vi "GetConfigChain.vi"(8 "error in (no error)":errorcluster, 11 "reference in":refnum<class "Frequency_Counter_BK.lvclass">) -> (0 "error out":errorcluster, 2 "Config out":string[](array[string]), 3 "reference out":refnum<class "Frequency_Counter_BK.lvclass">)   [LabVIEW 2022 SP3, in "Frequency_Counter_BK.lvlib" / "Frequency_Counter_BK.lvclass"]
uses:
  Frequency_Counter_BK.lvclass
  Components/Frequency_Counter_Base.lvlibp/Frequency_Counter_Base.lvclass
  Components/ViPER.lvlibp/ViPER.lvclass
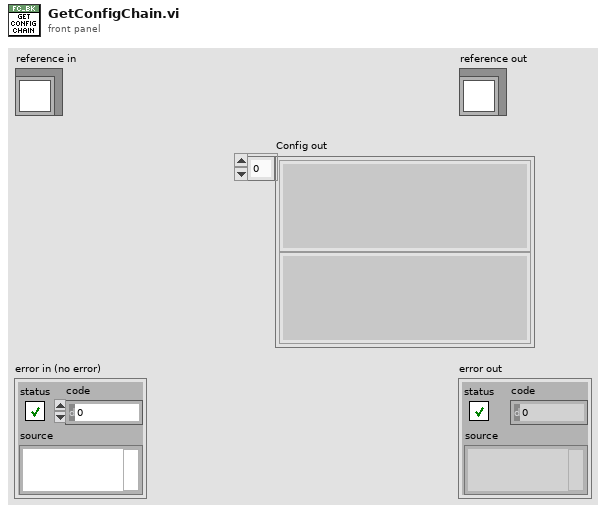
[diagram p1: front panel]
types:
  T1 = typedef "Frequency_Counter_BK.lvlib/Frequency_Counter_BK.lvclass/ObjectAttributes.ctl" = cluster{"Config":T2, "Freq":dbl}
  T2 = typedef "Frequency_Counter_BK.lvlib/Frequency_Counter_BK.lvclass/Config.ctl" = cluster{"ComPort":refnum<visa-resource-name>, "Function":i8, "Gate_Time":i8}
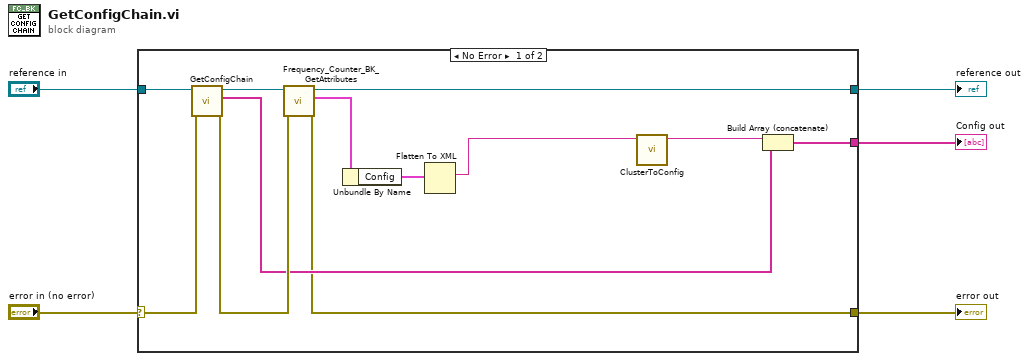
[diagram p0: block diagram]
diagram:
  n1 = case shown="No Error" "error in (no error)" {
    selector: "error in (no error)" -> [w13 w19]
    tunnel: [w6 w19] -> w4
    tunnel: [w11 w18] -> w2
    tunnel: "reference in" -> [w15 w18]
    tunnel: [w8 _] -> w1
    frame No Error {
      n2 = call-parent "GetConfigChain.vi"("error in (no error)"=w13, "reference in"=w15) -> ("error out"=w12:errorcluster, "Config out"=w9:string[], "reference out"=w14:refnum<class "Frequency_Counter_BK.lvclass">)  [unwired: 7 in]
      n3 = call "Frequency_Counter_BK_GetAttributes.vi"("error in (no error)"=w12, "reference in"=w14) -> ("error out"=w6:errorcluster, "Data"=w17:T1, "reference out"=w11:refnum<class "Frequency_Counter_BK.lvclass">)  [unwired: 6 in, 1 out]
      n4 = Unbundle By Name(w17) -> ("Config"=w16:T2)
      n5 = Flatten To XML(6:w16) -> (2:w7:string)
      n6 = call "ClusterToConfig.vi"("Cluster XML"=w7) -> ("Config XML"=w10:string)  [unwired: 10 in]
      n7 = Build Array (concatenate)(w10, w9) -> (w8:string[])
    }
    frame Error {
    }
  }
  "error out" <- w4
  "reference out" <- w2
  "Config out" <- w1
